vi "New_Sample_dialog.vi"(6 "Base Bath In":path) -> (0 "Notes About this Sample Out":string, 1 "Sample_name_out":string, 2 "Sample_data_base":path=path "/INL Macintosh/Users/timothymcjunkin/Desktop/diff_couple", 3 "Cancelled?":bool, 4 "Base Bath Out":path)   [LabVIEW 2011]
doc: "Pressing the New Sample button launches a warning message and then with user consent launches the dialog box. This dialog will guide the user through the process of creating a new sample. The base path will begin as the application path or another default. A folder of the same name as the Sample Name chosen will be created here. The OK button will be disabled until the user enters a non-blank sample name. Also, the OK button will be disabled if the user chooses a combination of a sample name and Base Path that already exists."
panel:
  out "appended path":path
  in  "Base Path":path
  in  "Notes About this Sample":string="Notes about your sample here"
  in  "Sample Name":string
  in  "Cancel":bool
  in  "OK":bool
  # "Enter a name and \nNotes about this new sample"
  # "Instructions:\n1. Select a Base Path (i.e.\n    starting directory)\n2. Type is a name for a \n    sample\n3. Hit OK\n\nHit cancel button to keep\nworking with current\nsample."
  # "Note Program will create\na directory with the\nsample name as a sub\ndirectory/folder beneath\nthe Base Path.\n\nThe main data file will\nbe <sample_name>_Main.xml\nin the created directory."
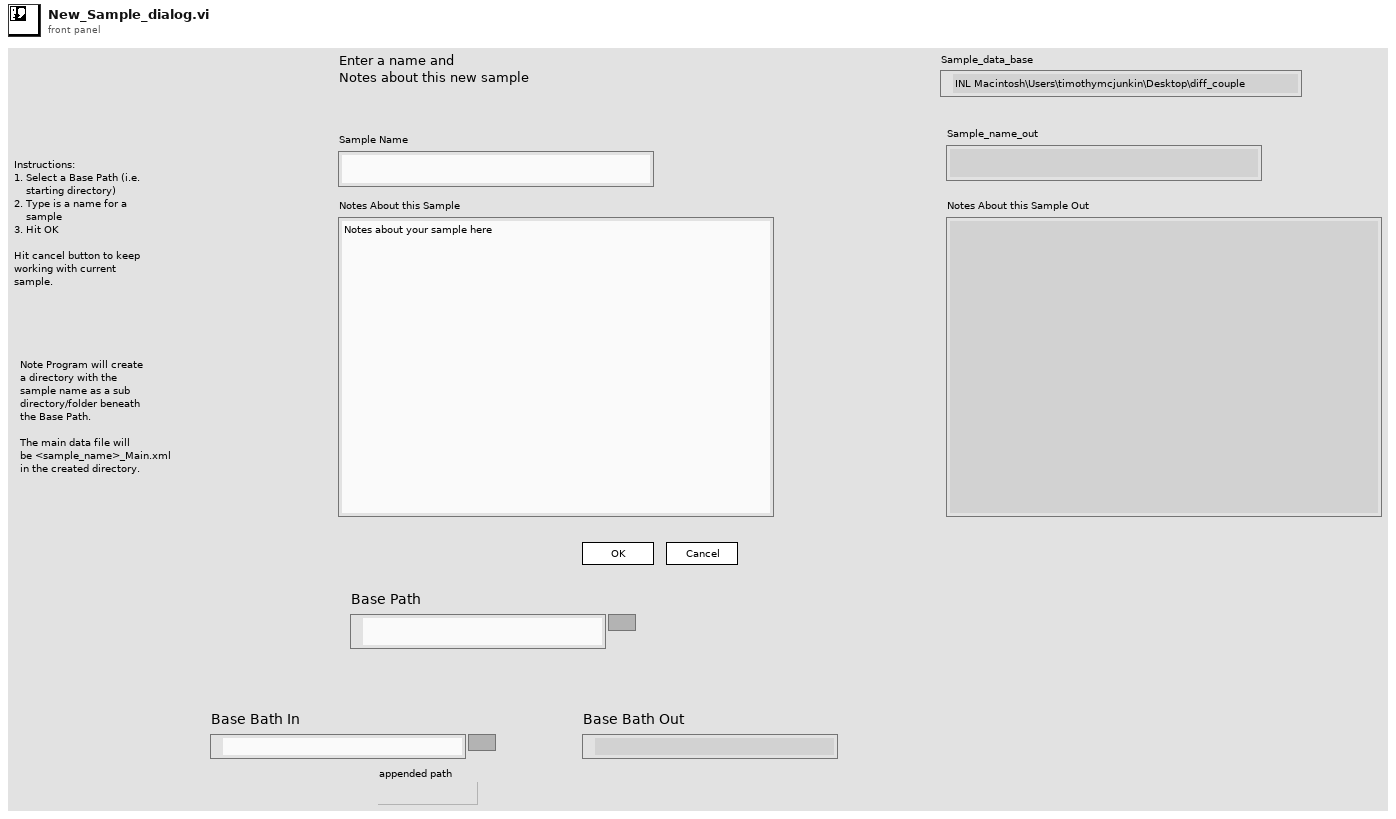
[diagram p1: front panel]
types:
  T1 = enum8{"Enabled", "Disabled", "Disabled and Grayed Out"}
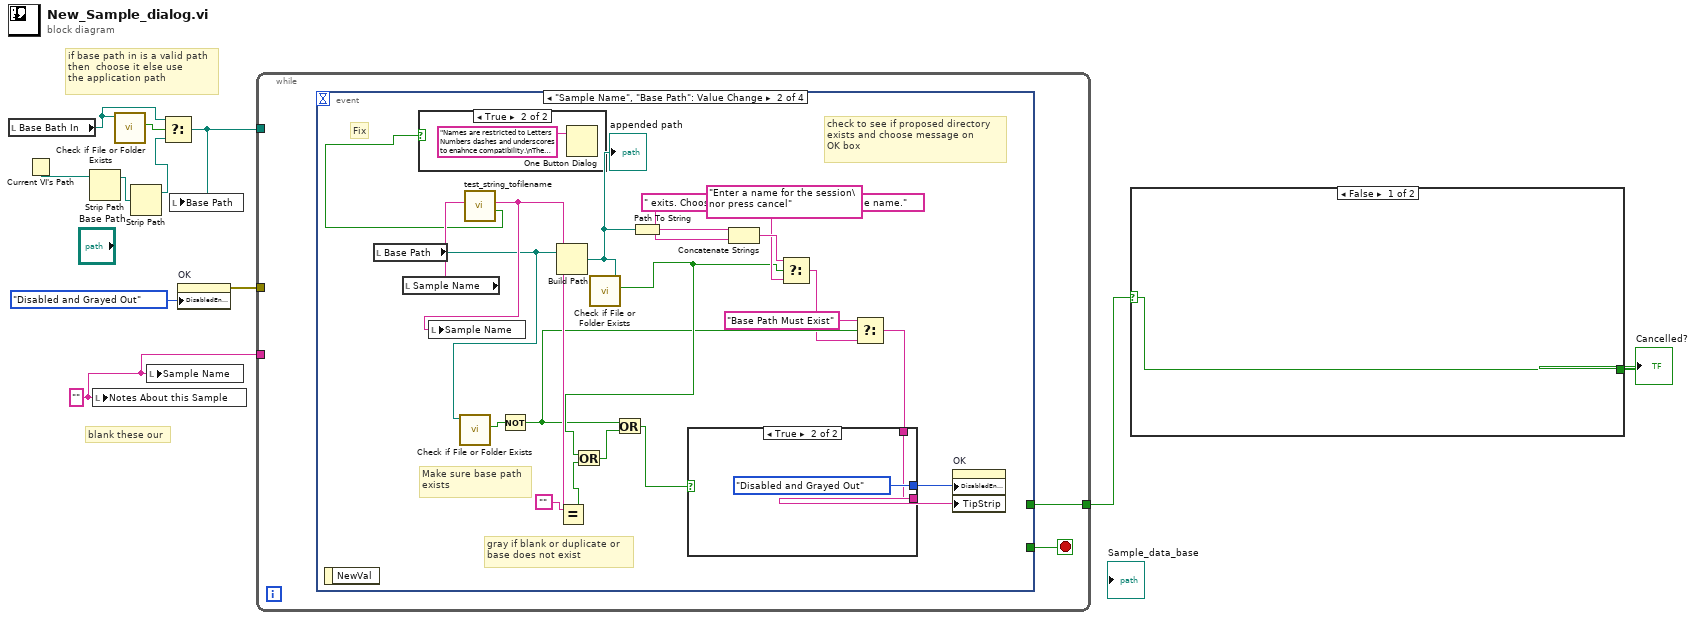
[diagram p0: block diagram]
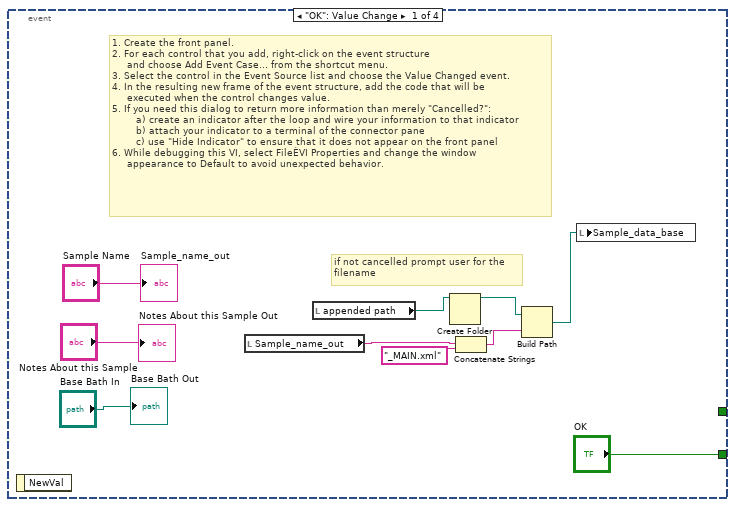
[diagram p3: hidden frame]
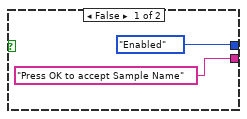
[diagram p5: hidden frame]
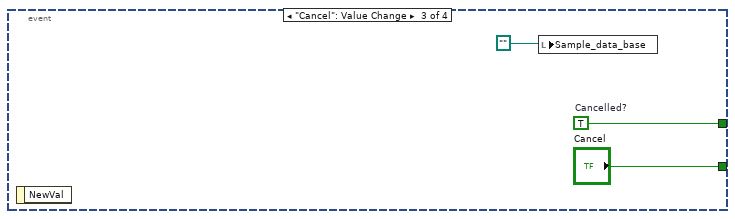
[diagram p6: hidden frame]
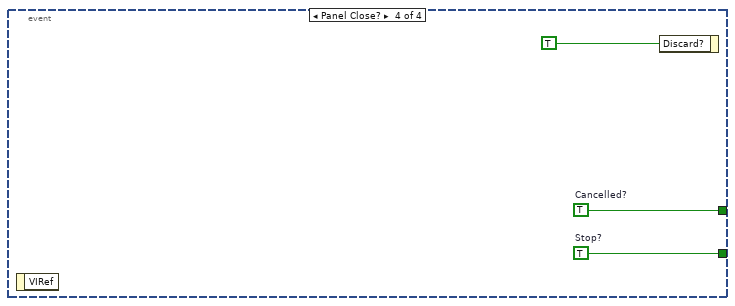
[diagram p7: hidden frame]
diagram:
  w9 = "" ("Notes About this Sample")
  # "if base path in is a valid path\nthen  choose it else use\nthe application path"
  # "blank these our"
  n1 = local read "Base Bath In"() -> (w6:path)
  n2 = Current VI's Path() -> (path=w4:path)
  n3 = Strip Path(path=w4) -> (stripped path=w3:path)  [unwired: 1 out]
  n4 = local write "Notes About this Sample"(w9) -> ()
  n5 = call <vilib>:"Check if File or Folder Exists.vi"("path"=w6) -> ("file or folder exists?"=w7:bool)  [unwired: 8 in, 2 out]
  n6 = Strip Path(path=w3) -> (stripped path=w2:path)  [unwired: 1 out]
  n7 = local write "Sample Name"(w9) -> ()
  n8 = Select(t=w6, s=w7, f=w2) -> (s? t:f=w5:path)
  n9 = local write "Base Path"(w5) -> ()
  n10 = property on="OK" class="Bool"("DisabledEnum"=T1."Disabled and Grayed Out" ("Disabled")) -> (error out=w1:errorcluster)  [unwired: 2 in, 1 out]
  n11 = while {
    tunnel: [w12] -> w11
    tunnel: w9 -> [_]
    tunnel: w5 -> [_]
    tunnel: w1 -> [_]
    stop <- w13 stop-if-true
    n12 = event shown="[1] \"Sample Name\", \"Base Path\": Value Change" {
      selector: _ -> [_ _ _ _]
      dyn-events: _ -> [_ _ _ _]
      timeout: _ -> [_ _ _ _]
      tunnel: ["OK" _ "Cancel" w54] -> w13
      tunnel: [_ _ w52 w53] -> w12
      event "OK": Value Change {
        # "if not cancelled prompt user for the\nfilename"
        # "1. Create the front panel.\n2. For each control that you add, right-click on the event structure \n     and choose Add Event Case... from the shortcut menu.\n3. Select the control in the Event Source list and choose the Value Changed event.\n4. In the resulting new frame of the event structure, add the code that will be \n     executed when the control changes value.\n5. If you need this dialog to return more information than merely \"Cancelled?\":\n        a) create an indicator after the loop and wire your information to that indicator\n        b) attach your indicator to a terminal of the connector pane\n        c) use \"Hide Indicator\" to ensure that it does not appear on the front panel\n6. While debugging this VI, select FileÈVI Properties and change the window \n     appearance to Default to avoid unexpected behavior."
        n13 = event-data() -> ()  [unwired: 1 in, 1 out]
        n14 = local read "Sample_name_out"() -> (w19:string)
        n15 = local read "appended path"() -> (w16:path)
        n16 = Create Folder(path (use dialog)=w16) -> (created path=w14:path)  [unwired: 2 in, 2 out]
        n17 = Concatenate Strings(w19, "_MAIN.xml" ("string")) -> (w17:string)
        n18 = Build Path(base path=w14, name or relative path=w17) -> (appended path=w15:path)
        n19 = local write "Sample_data_base"(w15) -> ()
        "Notes About this Sample Out" <- "Notes About this Sample"
        "Sample_name_out" <- "Sample Name"
        "Base Bath Out" <- "Base Bath In"
      }
      event "Sample Name", "Base Path": Value Change {
        # "gray if blank or duplicate or\nbase does not exist"
        # "Make sure base path\nexists"
        # "Fix"
        # "check to see if proposed directory\nexists and choose message on \nOK box"
        n20 = event-data() -> ()  [unwired: 1 in, 1 out]
        n21 = local read "Base Path"() -> (w32:path)
        n22 = local read "Sample Name"() -> (w35:string)
        n23 = call <vilib>:"Check if File or Folder Exists.vi"("path"=w32) -> ("file or folder exists?"=w31:bool)  [unwired: 8 in, 2 out]
        n24 = call "test_string_tofilename.vi"("Session Name/ID"=w35) -> ("fixed_name"=w34:bool, "CompliantName"=w33:string)  [unwired: 9 in]
        n25 = case shown="True" w34 {
          frame False {
          }
          frame True {
            n26 = One Button Dialog(message="Names are restricted to Letters Numbers dashes and underscores to enahnce compatibility.\nThe name entered has been modified Please check it.") -> ()  [unwired: 1 in, 1 out]
          }
        }
        n27 = local write "Sample Name"(w33) -> ()
        n28 = Not(x=w31) -> (.not. x?=w27:bool)
        n29 = Build Path(base path=w32, name or relative path=w33) -> (appended path=w40:path)
        "appended path" <- w40
        n30 = Equal?(x="", y=w33) -> (x = y?=w41:bool)
        n31 = call <vilib>:"Check if File or Folder Exists.vi"("path"=w40) -> ("file or folder exists?"=w30:bool)  [unwired: 8 in, 2 out]
        n32 = Or(x=w30, y=w41) -> (x .or. y?=w29:bool)
        n33 = Or(x=w27, y=w29) -> (x .or. y?=w28:bool)
        n34 = Path To String(path=w40) -> (string=w39:string)
        n35 = Concatenate Strings(w39, " exits. Choose a unique base path and sample name." ("string")) -> (w37:string)
        n36 = Select(t=w37, s=w30, f="Enter a name for the session\nor press cancel" ("Tip Strip")) -> (s? t:f=w26:string)
        n37 = Select(t="Base Path Must Exist", s=w27, f=w26) -> (s? t:f=w24:string)
        n38 = case shown="True" w28 {
          tunnel: [T1."Enabled" ("Disabled") T1."Disabled and Grayed Out" ("Disabled")] -> w43
          tunnel: ["Press OK to accept Sample Name" ("Tip Strip") w48] -> w42
          tunnel: w24 -> [_ w48]
          frame False {
          }
          frame True {
          }
        }
        n39 = property on="OK" class="Bool"("DisabledEnum"=w43, "TipStrip"=w42) -> ()  [unwired: 2 in, 2 out]
      }
      event "Cancel": Value Change {
        w52 = TRUE  # Cancelled?
        n40 = event-data() -> ()  [unwired: 1 in, 1 out]
        n41 = local write "Sample_data_base"(path "") -> ()
      }
      event Panel Close? {
        w53 = TRUE  # Cancelled?
        w54 = TRUE  # Stop?
        n42 = event-data() -> ()  [unwired: 1 in, 1 out]
        n43 = event-data("Discard?"=TRUE) -> ()  [unwired: 1 in, 1 out]
      }
    }
  }
  n44 = case shown="False" w11 {
    selector: w11 -> [w56 w57]
    tunnel: [w56 w57] -> w10
    frame False {
    }
    frame True {
    }
  }
  "Cancelled?" <- w10
